vi "Get 664 Message Data.vi"(0 "MSG DATA":u8[](array[numeric]) format="%.0x", 5 "664 Parameter":T1, 11 "error in (no error)":errorcluster) -> (4 "Value":dbl format="%#_10g", 15 "error out":errorcluster)   [LabVIEW 2015, in "AIT 664 Custom Device.lvlib"]
uses:
  AIT 664 Custom Device.lvlib
  Controls/664 -Param.ctl
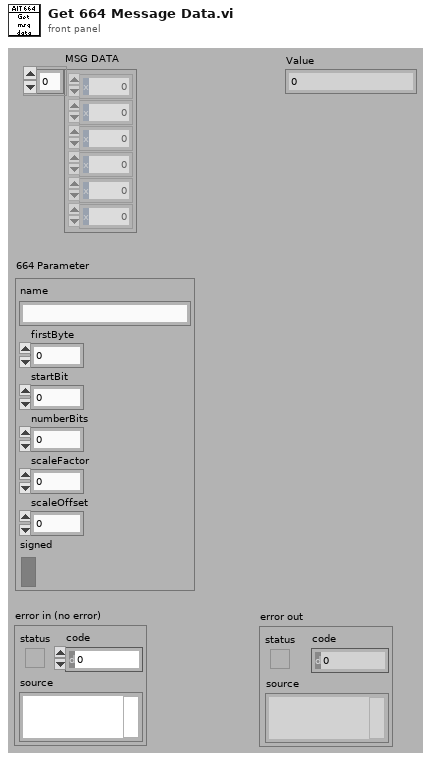
[diagram p1: front panel]
types:
  T1 = typedef "AIT 664 Custom Device.lvlib/664 -Param.ctl" = cluster{"name":string, "firstByte":i32, "startBit":i32, "numberBits":i32, "scaleFactor":dbl, "scaleOffset":dbl, "signed":bool}
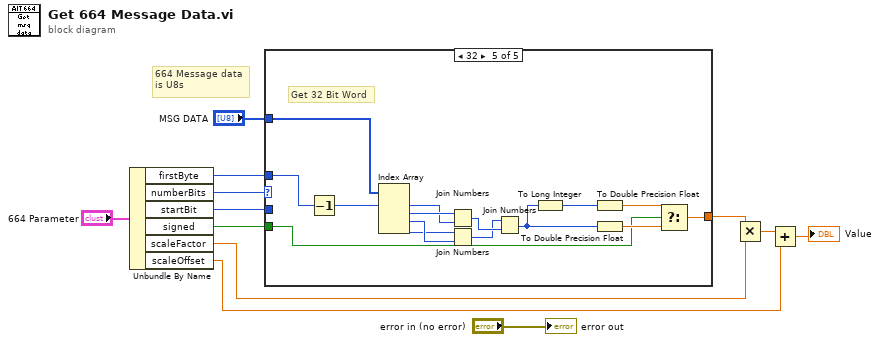
[diagram p0: block diagram]
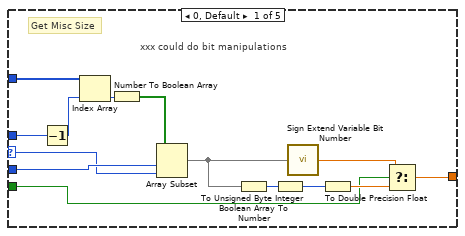
[diagram p2: hidden frame]
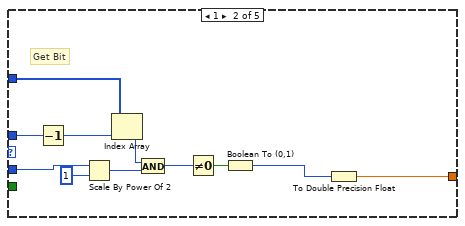
[diagram p3: hidden frame]
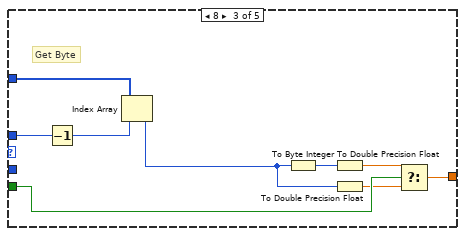
[diagram p4: hidden frame]
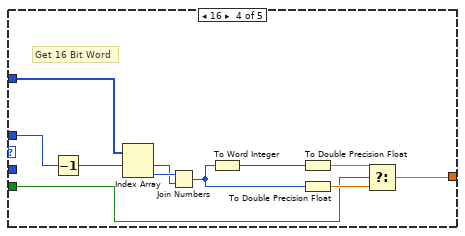
[diagram p5: hidden frame]
diagram:
  # "664 Message data\nis U8s"
  n1 = Unbundle By Name("664 Parameter") -> ("firstByte"=w9:i32, "numberBits"=w8:i32, "startBit"=w7:i32, "signed"=w2:bool, "scaleFactor"=w5:dbl, "scaleOffset"=w4:dbl)
  n2 = case shown="32" w8 {
    selector: w8 -> [w20 _ _ _ _]
    tunnel: "MSG DATA" -> [w24 w36 w46 w56 w70]
    tunnel: w9 -> [w26 w37 w45 w57 w72]
    tunnel: w7 -> [w21 w30 _ _ _]
    tunnel: w2 -> [w17 _ w42 w50 w64]
    tunnel: [w16 w27 w39 w52 w65] -> w1
    frame 0, Default {
      # "xxx could do bit manipulations"
      # "Get Misc Size"
      n3 = Decrement(x=w26) -> (x-1=w23:i32)
      n4 = Index Array(array=w24, index=w23) -> (element=w25:u8)
      n5 = Number To Boolean Array(number=w25) -> (Boolean array=w22:bool[])
      n6 = Array Subset(array=w22, index=w21, length=w20) -> (w14:bool[])
      n7 = Boolean Array To Number(Boolean array=w14) -> (number=w15:u32)
      n8 = To Unsigned Byte Integer(number=w15) -> (unsigned 8bit integer=w18:u8)
      n9 = call "Sign Extend Variable Bit Number.vi"("Variable Bit Number"=w14) -> ("Sign extended value"=w13:dbl)  [unwired: 14 in]
      n10 = To Double Precision Float(number=w18) -> (double precision float=w19:dbl)
      n11 = Select(t=w13, s=w17, f=w19) -> (s? t:f=w16:dbl)
    }
    frame 1 {
      # "Get Bit"
      n12 = Decrement(x=w37) -> (x-1=w33:i32)
      n13 = Scale By Power Of 2(n=w30, x=u8 1) -> (x*2^n=w35:u8)
      n14 = Index Array(array=w36, index=w33) -> (element=w34:u8)
      n15 = And(x=w34, y=w35) -> (x .and. y?=w29:u8)
      n16 = Not Equal To 0?(x=w29) -> (x != 0?=w31:bool)
      n17 = Boolean To (0,1)(Boolean=w31) -> (0, 1=w28:i16)
      n18 = To Double Precision Float(number=w28) -> (double precision float=w27:dbl)
    }
    frame 8 {
      # "Get Byte"
      n19 = Decrement(x=w45) -> (x-1=w44:i32)
      n20 = Index Array(array=w46, index=w44) -> (element=w38:u8)
      n21 = To Byte Integer(number=w38) -> (8bit integer=w43:i8)
      n22 = To Double Precision Float(number=w43) -> (double precision float=w41:dbl)
      n23 = To Double Precision Float(number=w38) -> (double precision float=w40:dbl)
      n24 = Select(t=w41, s=w42, f=w40) -> (s? t:f=w39:dbl)
    }
    frame 16 {
      # "Get 16 Bit Word"
      n25 = Decrement(x=w57) -> (x-1=w55:i32)
      n26 = Index Array(array=w56, index #1=w55) -> (element #1=w48:u8, element #2=w49:u8)  [unwired: 1 in]
      n27 = Join Numbers(hi=w49, lo=w48) -> ((hi.lo)=w47:u16)
      n28 = To Word Integer(number=w47) -> (16bit integer=w51:i16)
      n29 = To Double Precision Float(number=w51) -> (double precision float=w54:dbl)
      n30 = To Double Precision Float(number=w47) -> (double precision float=w53:dbl)
      n31 = Select(t=w54, s=w50, f=w53) -> (s? t:f=w52:dbl)
    }
    frame 32 {
      # "Get 32 Bit Word"
      n32 = Decrement(x=w72) -> (x-1=w71:i32)
      n33 = Index Array(array=w70, index #1=w71) -> (element #1=w68:u8, element #2=w69:u8, element #3=w62:u8, element #4=w61:u8)  [unwired: 3 in]
      n34 = Join Numbers(hi=w69, lo=w68) -> ((hi.lo)=w60:u16)
      n35 = Join Numbers(hi=w61, lo=w62) -> ((hi.lo)=w59:u16)
      n36 = Join Numbers(hi=w59, lo=w60) -> ((hi.lo)=w58:u32)
      n37 = To Long Integer(number=w58) -> (32bit integer=w63:i32)
      n38 = To Double Precision Float(number=w63) -> (double precision float=w67:dbl)
      n39 = To Double Precision Float(number=w58) -> (double precision float=w66:dbl)
      n40 = Select(t=w67, s=w64, f=w66) -> (s? t:f=w65:dbl)
    }
  }
  n41 = Multiply(x=w1, y=w5) -> (x*y=w6:dbl)
  n42 = Add(x=w6, y=w4) -> (x+y=→"Value":dbl)
  "error out" <- "error in (no error)"
